vi "Start Cooking Recipe.vi"(8 "error in (no error)":errorcluster, 10 "Steps":refnum<class "Recipe Step.lvclass">[](array[class]), 11 "Cooker Actor in":refnum<class "Cooker Actor.lvclass">) -> (0 "error out":errorcluster, 3 "Cooker Actor out":refnum<class "Cooker Actor.lvclass">)   [LabVIEW 2024, in "Cooker Actor.lvlib" / "Cooker Actor.lvclass"]
uses:
  Cooker Actor.lvclass
  Support/Recipe Step/Recipe Step.lvclass
  Cooker Actor.lvclass/Cooker Actor.ctl
  Support/Recipe/Recipe.lvclass
  <vilib>/ActorFramework/Actor/Actor.lvclass
  Kitchen Messaging Interface/Kitchen Messaging Interface Messages/Dye Recipe Table Step by Index Msg/Dye Recipe Table Step by Index Msg.lvclass
  C:/Program Files/National Instruments/LabVIEW 2024/vi.lib/ActorFramework/Actor/Actor.lvclass
  C:/Users/burakkorkmaz/Desktop/Leveling/repo/Cooker Actor/Cooker Actor/Cooker Actor.lvclass
  C:/Users/burakkorkmaz/Desktop/Leveling/repo/Cooker Messaging Interface/Cooker Messaging Interface/Cooker Messaging Interface.lvclass
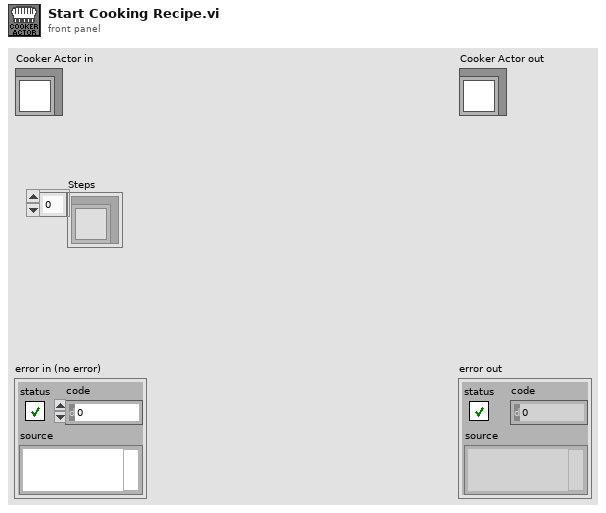
[diagram p1: front panel]
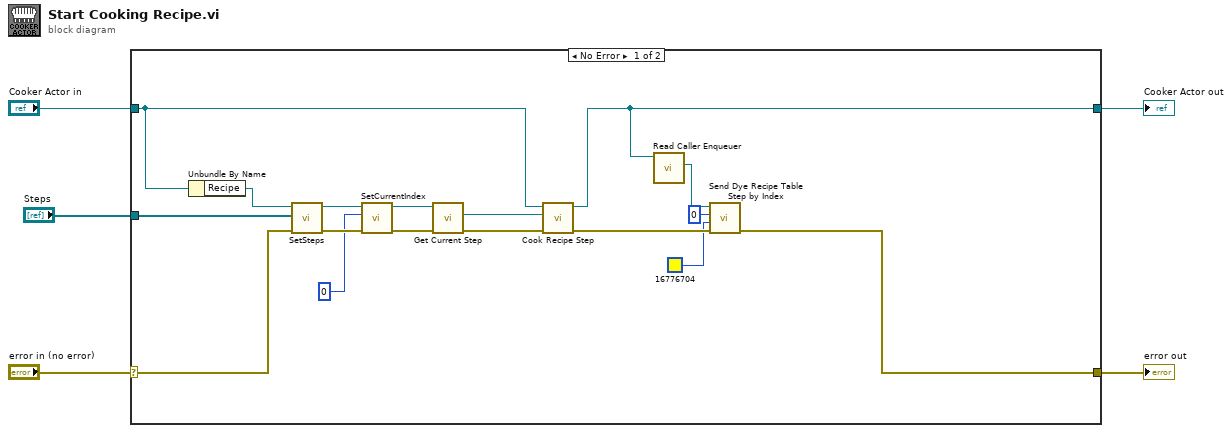
[diagram p0: block diagram]
diagram:
  n1 = case shown="No Error" "error in (no error)" {
    selector: "error in (no error)" -> [w18 w24]
    tunnel: [w9 w24] -> w4
    tunnel: [w10 w23] -> w2
    tunnel: "Cooker Actor in" -> [w15 w23]
    tunnel: "Steps" -> [w21 _]
    frame No Error {
      n2 = Unbundle By Name(w15) -> ("Recipe"=w22:refnum<class "Recipe.lvclass">)
      n3 = call-dynamic "SetSteps.vi"("Error In"=w18, "Steps"=w21, "reference in"=w22) -> ("Error Out"=w20:errorcluster, "reference out"=w13:refnum<class "Recipe.lvclass">)  [unwired: 7 in]
      n4 = call-dynamic "SetCurrentIndex.vi"("Error In"=w20, "Current Index"=u64 0, "reference in"=w13) -> ("Error Out"=w14:errorcluster, "reference out"=w12:refnum<class "Recipe.lvclass">)  [unwired: 7 in]
      n5 = call-dynamic "Get Current Step.vi"("error in (no error)"=w14, "Recipe in"=w12) -> ("error out"=w19:errorcluster, "Recipe Step"=w16:refnum<class "Recipe Step.lvclass">)  [unwired: 7 in, 1 out]
      n6 = call-dynamic "Cook Recipe Step.vi"("error in (no error)"=w19, "Recipe Step"=w16, "Cooker Actor in"=w15) -> ("error out"=w17:errorcluster, "Cooker Actor out"=w10:refnum<class "Cooker Actor.lvclass">)  [unwired: 7 in]
      n7 = call <vilib>:"Read Caller Enqueuer.vi"("Actor"=w10) -> ("Caller Enqueuer"=w8:refnum<class "Message Enqueuer.lvclass">)  [unwired: 10 in]
      n8 = call "Send Dye Recipe Table Step by Index.vi"("error in (no error)"=w17, "Dye Color"=u32 16776704, "Index"=u64 0, "Message Enqueuer"=w8) -> ("error out"=w9:errorcluster)  [unwired: 6 in, 1 out]
    }
    frame Error {
    }
  }
  "error out" <- w4
  "Cooker Actor out" <- w2
